vi "Open DB Ref.vi"(8 "error in (no error)":errorcluster, 10 "DAQ Type":enum16{"Hardware", "Simulation"}(ring), 11 "Access in":refnum<class "Access.lvclass">) -> (0 "error out":errorcluster, 3 "Access out":refnum<class "Access.lvclass">)   [LabVIEW 2021, in "Database.lvlib" / "Access.lvclass"]
uses:
  Access.lvclass
  Access.lvclass/Access.ctl
  Database.lvlib
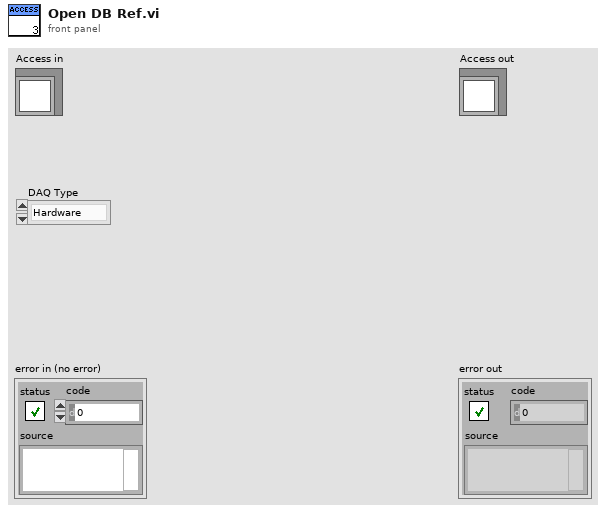
[diagram p1: front panel]
types:
  T1 = typedef "NI_Database_API.lvlib/Conn ObjectReference.ctl" = refnum<k1>
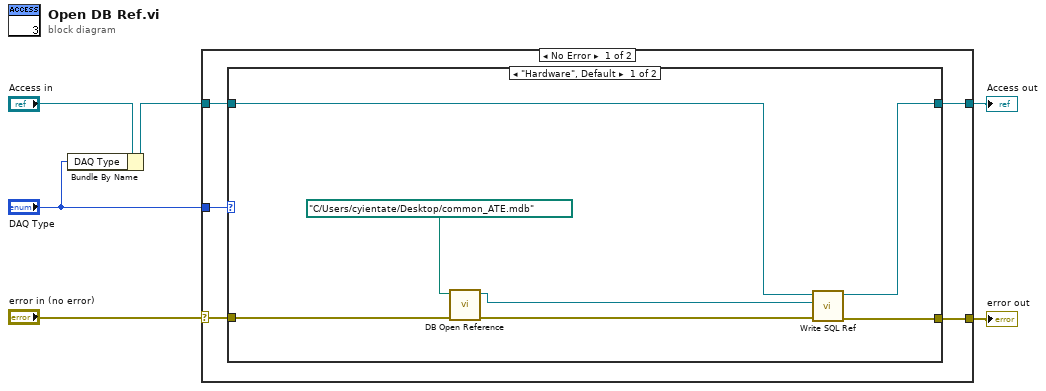
[diagram p0: block diagram]
diagram:
  n1 = Bundle By Name(cluster="Access in", "DAQ Type"="DAQ Type") -> (w2:refnum<class "Access.lvclass">)
  n2 = case shown="No Error" "error in (no error)" {
    selector: "error in (no error)" -> [w8 w21]
    tunnel: [w10 w22] -> w5
    tunnel: w2 -> [w9 w22]
    tunnel: [w11 w21] -> w3
    tunnel: "DAQ Type" -> [w7 _]
    frame No Error {
      n3 = case shown="\"Hardware\", Default" w7 {
        tunnel: [w18 w19] -> w11
        tunnel: [w17 w20] -> w10
        tunnel: w9 -> [w16 w20]
        tunnel: w8 -> [w15 w19]
        frame "Hardware", Default {
          n4 = call "DB Open Reference.vi"("error in (no error)"=w15, "Database Path"=path "C:/Users/cyientate/Desktop/common_ATE.mdb") -> ("error out"=w14:errorcluster, "connection reference"=w13:T1)  [unwired: 8 in]
          n5 = call-dynamic "Write SQL Ref.vi"("error in (no error)"=w14, "connection reference"=w13, "Access in"=w16) -> ("error out"=w18:errorcluster, "Access out"=w17:refnum<class "Access.lvclass">)  [unwired: 7 in]
        }
        frame "Simulation" {
        }
      }
    }
    frame Error {
    }
  }
  "error out" <- w3
  "Access out" <- w5
